vi "DB Update Data(Feedback).vi"(4 "Pos":cluster{"index":i32, "Len":i32}, 5 "condtinal":string, 6 "Sel index":i32, 7 "data":variant, 8 "error in (no error)":errorcluster caption="错误输入（无错误）", 9 "Code":string, 10 "table":string, 11 "Connncet State":T1) -> (0 "error out":errorcluster caption="错误输出", 2 "State":bool, 3 "Connncet State out":T1)   [LabVIEW 2014]
uses:
  <vilib>/addons/database/NI_Database_API.lvlib
  Ctr/Constr.ctl
  <vilib>/addons/database/Connection.llb/Conn ObjectReference.ctl
  Ctr/Conneect State.ctl
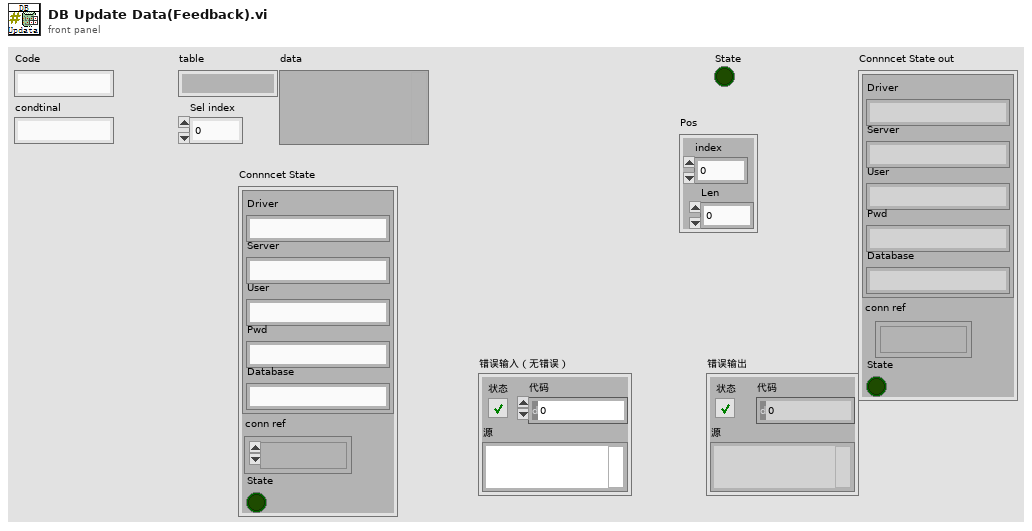
[diagram p1: front panel]
types:
  T1 = typedef "Conneect State.ctl" = cluster{"Constr":T2, "conn ref":T3, "State":bool}
  T2 = typedef "Constr.ctl" = cluster{"Driver":string, "Server":string, "User":string, "Pwd":string, "Database":string}
  T3 = typedef "NI_Database_API.lvlib/Conn ObjectReference.ctl" = refnum<k1>
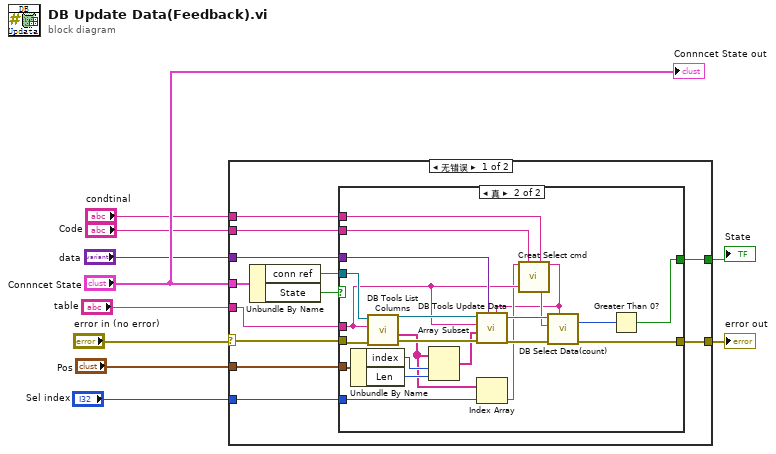
[diagram p0: block diagram]
diagram:
  n1 = case shown="无错误" "error in (no error)" {
    selector: "error in (no error)" -> [w21 w45]
    tunnel: "Connncet State" -> [w22 _]
    tunnel: "table" -> [w18 _]
    tunnel: "data" -> [w17 _]
    tunnel: "Pos" -> [w16 _]
    tunnel: "Sel index" -> [w15 _]
    tunnel: [w14 w45] -> w4
    tunnel: [w13 _] -> w3
    tunnel: "Code" -> [w12 _]
    tunnel: "condtinal" -> [w11 _]
    frame No Error {
      n2 = Unbundle By Name(w22) -> ("conn ref"=w19:T3, "State"=w20:bool)
      n3 = case shown="真" w20 {
        tunnel: w21 -> [w23 w44]
        tunnel: w19 -> [_ w43]
        tunnel: w18 -> [_ w33]
        tunnel: w17 -> [_ w40]
        tunnel: w16 -> [_ w38]
        tunnel: w15 -> [_ w30]
        tunnel: [w23 w29] -> w14
        tunnel: [_ w26] -> w13
        tunnel: w12 -> [_ w28]
        tunnel: w11 -> [_ w25]
        frame False {
        }
        frame True {
          n4 = Unbundle By Name(w38) -> ("index"=w37:i32, "Len"=w36:i32)
          n5 = call <vilib>:"DB Tools List Columns.vi"("error in (no error)"=w44, "table"=w33, "connection reference"=w43) -> ("error out"=w42:errorcluster, "columns"=w32:string[], "connection reference out"=w41:T3)  [unwired: 1 in, 1 out]
          n6 = Array Subset(array=w32, index=w37, length=w36) -> (w39:string[])
          n7 = Index Array(array=w32, index=w30) -> (element=w31:string)
          n8 = call "Creat Select cmd.vi"("Col"=w31, "Code"=w28, "Condtion"=w25) -> ("Str"=w24:string)  [unwired: 11 in, 1 out]
          n9 = call <vilib>:"DB Tools Update Data.vi"("condition"=w24, "data"=w40, "error in (no error)"=w42, "columns"=w39, "table"=w33, "connection reference"=w41) -> ("error out"=w35:errorcluster, "connection reference out"=w34:T3)  [unwired: 4 in]
          n10 = call "DB Select Data(count).vi"("condition"=w24, "error in (no error)"=w35, "table"=w33, "connection reference"=w34) -> ("error out"=w29:errorcluster, "Count"=w27:i32)  [unwired: 5 in, 1 out]
          n11 = Greater Than 0?(x=w27) -> (x > 0?=w26:bool)
        }
      }
    }
    frame Error {
    }
  }
  "error out" <- w4
  "State" <- w3
  "Connncet State out" <- "Connncet State"
